vi "Constants.vi"() -> ()   [LabVIEW 2027, in "System Monitor Shared.lvlib"]
doc: "Use this Global VI to access the GUIDs assigned to the page resources of the Custom Device."
uses:
  System Monitor Shared.lvlib
panel:
  in  "Tab Control":enum32{"GUIDS", "Constants", "Properties"}(tab)=enum."Properties"
  in  "Advanced":string="85f74618-51ce-4e99-a8ac-e21873927867"
  in  "System Monitor":string="9c57ba26-991c-43a0-bc8f-8fe20f3ab37d"
  in  "Incoming":string="Incoming"
  in  "Update Rate (Hz)":string="Update Rate (Hz)"
  in  "Number of CPU Cores":string="Number of CPU Cores"
  in  "Compiled.Settings":string="Compiled.Settings"
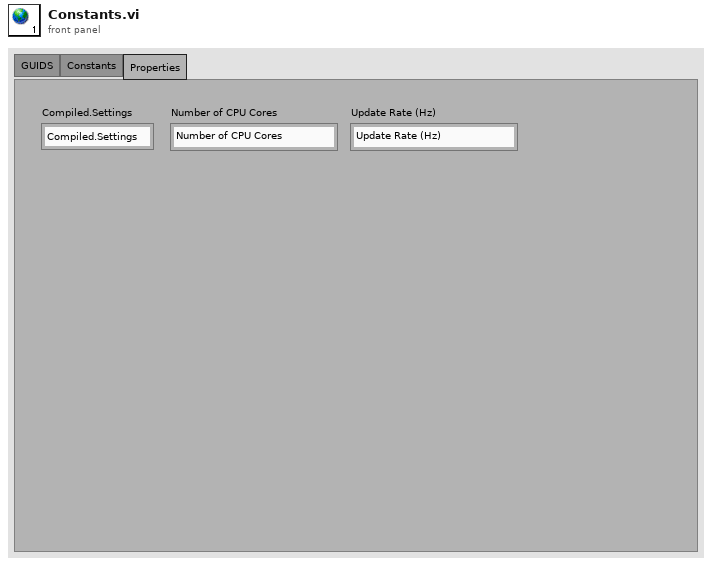
[diagram p1: front panel]
diagram:
